vi "Complex Exponential Signal.vi"(5 "offset":dbl format="%0.2p", 6 "sampling info":cluster{"Fs":dbl, "#s":dbl}={"Fs"=1000.0, "#s"=1000.0} {"Fs" format="%.2p"}, 8 "error in (no error)":errorcluster, 10 "amplitude":cdb=1.0+0.0i format="%0.2p", 11 "frequency":dbl=10.0 format="%0.2p") -> (0 "error out":errorcluster, 3 "signal out":waveform(cdb))   [LabVIEW 2019]
uses:
  <vilib>/Analysis/1siggen.llb/Ramp Pattern by Samples.vi
  <vilib>/Analysis/NI_AALBase.lvlib
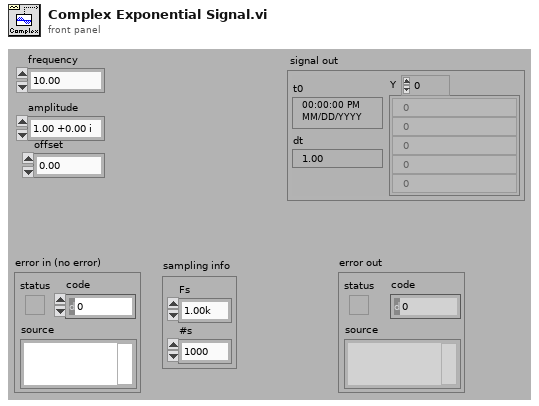
[diagram p1: front panel]
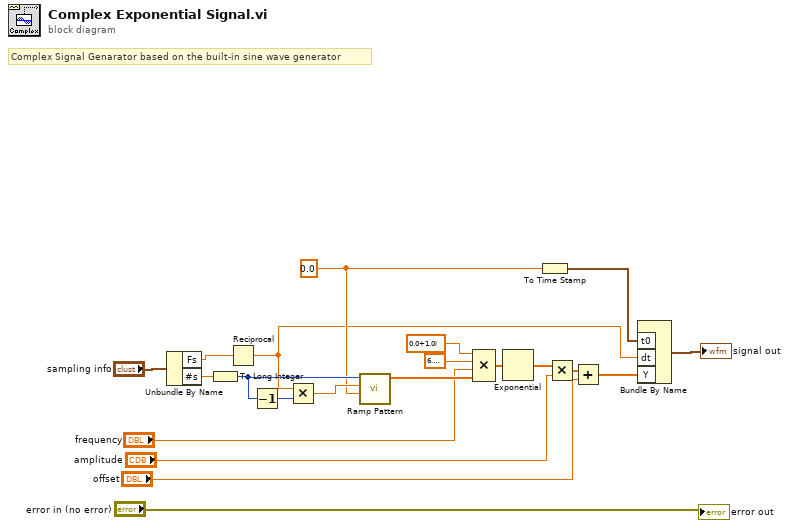
[diagram p0: block diagram]
diagram:
  w15 = 0.0 ("start")
  # "Complex Signal Genarator based on the built-in sine wave generator"
  n1 = Unbundle By Name("sampling info") -> ("Fs"=w2:dbl, "#s"=w20:dbl)
  n2 = To Long Integer(number=w20) -> (32bit integer=w19:i32)
  n3 = Reciprocal(x=w2) -> (1/x=w13:dbl)
  n4 = Decrement(x=w19) -> (x-1=w18:i32)
  n5 = Multiply(x=w13, y=w18) -> (x*y=w17:dbl)
  n6 = call-poly <vilib>:"Ramp Pattern.vi"("start"=w15, "end"=w17, "samples"=w19) -> ("Ramp Pattern"=w16:dbl[])  [unwired: 7 in, 1 out]
  n7 = Compound Arithmetic op=MULTIPLY(cdb 0.0+1.0i ("value"), 6.283185307179586, "frequency", w16) -> (w8:cdb[])
  n8 = Exponential(1:w8) -> (0:w11:cdb[])
  n9 = To Time Stamp(1:w15) -> (0:w14:timestamp)
  n10 = Multiply(x=w11, y="amplitude") -> (x*y=w10:cdb[])
  n11 = Add(x=w10, y="offset") -> (x+y=w5:cdb[])
  n12 = Bundle By Name("t0"=w14, "dt"=w13, "Y"=w5) -> (→"signal out":waveform(cdb))  [unwired: 1 in]
  "error out" <- "error in (no error)"
